vi "Process_Output.vi"(0 "Data string":string, 5 "Table reference":refnum<vi>, 11 "Error In":errorcluster) -> (4 "R":u16, 6 "G":u16, 8 "B":u16, 10 "Unfiltered":u16, 15 "Error Out":errorcluster)   [LabVIEW 2018]
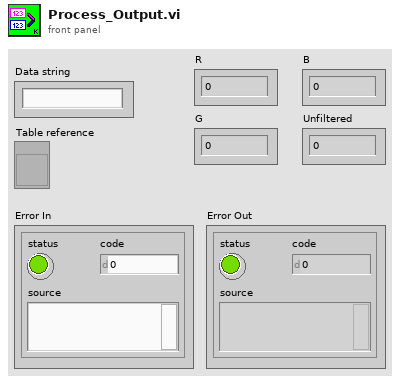
[diagram p1: front panel]
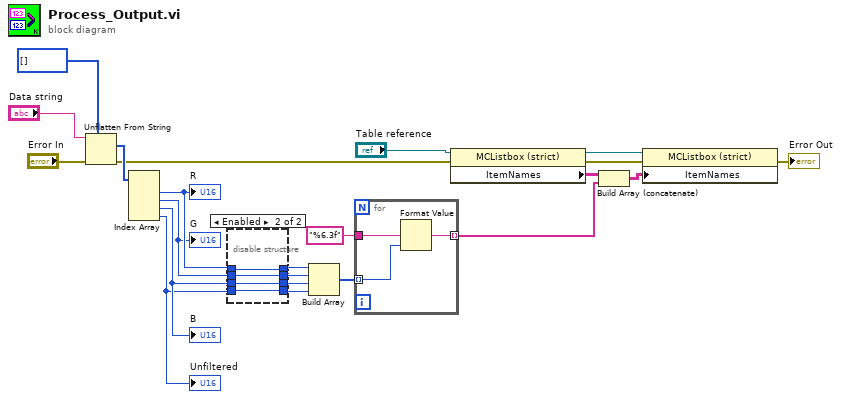
[diagram p0: block diagram]
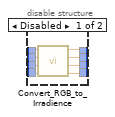
[diagram p2: hidden frame]
diagram:
  n1 = Unflatten From String(type=u16[] [], binary string="Data string", error in (no error)="Error In") -> (value=w21:u16[], error out=w17:errorcluster)  [unwired: 2 in, 1 out]
  n2 = Index Array(array=w21) -> (element #1=w4:u16, element #2=w3:u16, element #3=w2:u16, element #4=w1:u16)  [unwired: 4 in]
  "R" <- w4
  "G" <- w3
  "B" <- w2
  "Unfiltered" <- w1
  n3 = disable-structure shown="Enabled" {
    disable-tunnel: [w30 w34] -> w15
    disable-tunnel: [w29 w33] -> w14
    disable-tunnel: [w28 w32] -> w13
    disable-tunnel: [w27 w31] -> w12
    disable-tunnel: w4 -> [w26 w34]
    disable-tunnel: w3 -> [w25 w33]
    disable-tunnel: w2 -> [w24 w32]
    disable-tunnel: w1 -> [w23 w31]
    frame Disabled {
      n4 = call "Convert_RGB_to_Irradience.vi"("Unfiltered"=w23, "B"=w24, "G"=w25, "R"=w26) -> ("Unfiltered"=w27:dbl, "B"=w28:dbl, "G"=w29:dbl, "R"=w30:dbl)  [unwired: 4 in]
    }
    frame Enabled {
    }
  }
  n5 = Build Array(w15, w14, w13, w12) -> (w11:u16[])
  n6 = for {
    tunnel: "%6.3f" ("format string") -> [w37]
    tunnel: w11 -> [w36] mode=indexing
    tunnel: [w35] -> w9 mode=indexing
    n7 = Format Value(format string=w37, value (0)=w36) -> (output string=w35:string)  [unwired: 1 in]
  }
  n8 = property class="MCListbox (strict)"(reference="Table reference", error in=w17) -> (reference out=w8:refnum<vi>, error out=w7:errorcluster, "ItemNames"=w10:string[][])
  n9 = Build Array (concatenate)(w10, w9) -> (w6:string[][])
  n10 = property class="MCListbox (strict)"(reference=w8, error in=w7, "ItemNames"=w6) -> (error out=→"Error Out":errorcluster)  [unwired: 1 out]
